vi "Untitled 2.vi"() -> ()   [LabVIEW 2016]
panel:
  out "Packet OK?":bool
  out "Data Out 2":string
  in  "Packet Length":i32
  in  "Data Out":string
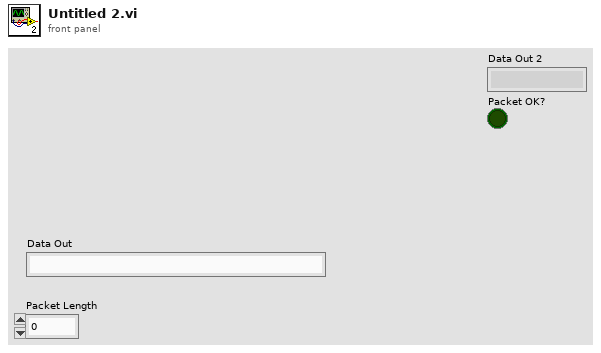
[diagram p1: front panel]
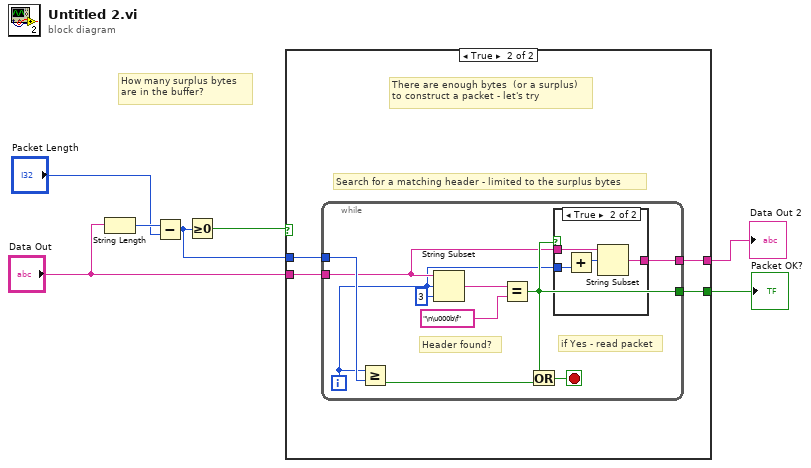
[diagram p0: block diagram]
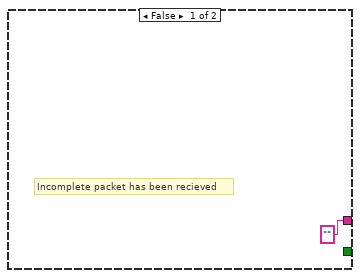
[diagram p2: hidden frame]
diagram:
  # "How many surplus bytes\nare in the buffer?"
  n1 = String Length(string="Data Out") -> (length=w5:i32)
  n2 = Subtract(x=w5, y="Packet Length") -> (x-y=w2:i32)
  n3 = Greater Or Equal To 0?(x=w2) -> (x >= 0?=w3:bool)
  n4 = case shown="True" w3 {
    tunnel: "Data Out" -> [_ w12]
    tunnel: ["" ("Data Out") w9] -> w6
    tunnel: w2 -> [_ w11]
    tunnel: [_ w10] -> w1
    frame False {
      # "Incomplete packet has been recieved"
    }
    frame True {
      # "Search for a matching header - limited to the surplus bytes"
      # "There are enough bytes  (or a surplus)\nto construct a packet - let's try"
      n5 = while {
        tunnel: w12 -> [w14]
        tunnel: w11 -> [w21]
        tunnel: [w16] -> w10
        tunnel: [w15] -> w9
        i -> [w13]
        stop <- w20 stop-if-true
        # "if Yes - read packet"
        # "Header found?"
        n6 = Greater Or Equal?(x=w13, y=w21) -> (x >= y?=w19:bool)
        n7 = String Subset(string=w14, offset (0)=w13, length (rest)=3 ("length (rest)")) -> (substring=w18:string)
        n8 = Equal?(x=w18, y="\n\u000b\f") -> (x = y?=w16:bool)
        n9 = Or(x=w16, y=w19) -> (x .or. y?=w20:bool)
        n10 = case shown="True" w16 {
          tunnel: [_ w26] -> w15
          tunnel: w14 -> [_ w25]
          tunnel: w13 -> [_ w23]
          frame False {
          }
          frame True {
            n11 = Add(y=w23) -> (x+y=w24:i32)  [unwired: 1 in]
            n12 = String Subset(string=w25, offset (0)=w24) -> (substring=w26:string)  [unwired: 1 in]
          }
        }
      }
    }
  }
  "Data Out 2" <- w6
  "Packet OK?" <- w1
